vi "ir test.vi"   [LabVIEW 2012, in "Testing.lvrbt"]
uses:
  Testing.lvrbt
  <vilib>/NXT/HiTechnic/HiTechnic Controls/HiTechnic Port.ctl
  <vilib>/NXT/Block Support/NXT_InputPort.ctl
  <vilib>/NXT/Block Support/NXT_ButtonSelector.ctl
  <vilib>/NXT/Dual Mode Library/Sensors/readNXTButton.vi
  <vilib>/NXT/Dual Mode Library/Waits/Wait_Num.vi
  <vilib>/NXT/Dual Mode Library/Display/drawNumber.vi
types:
  T1 = typedef "HiTechnic Port.ctl" = cluster{"Port":T2, "MUX Port":u8}
  T2 = typedef "NXT_InputPort.ctl" = u32
  T3 = typedef "NXT_ButtonSelector.ctl" = u16
  T4 = cluster{"Direction (0-9)":i16, "Signal Strength (Array)":u8[]}
  T5 = typedef "LVHSConnector.ctl" = refnum<class "BrickReference.lvclass">
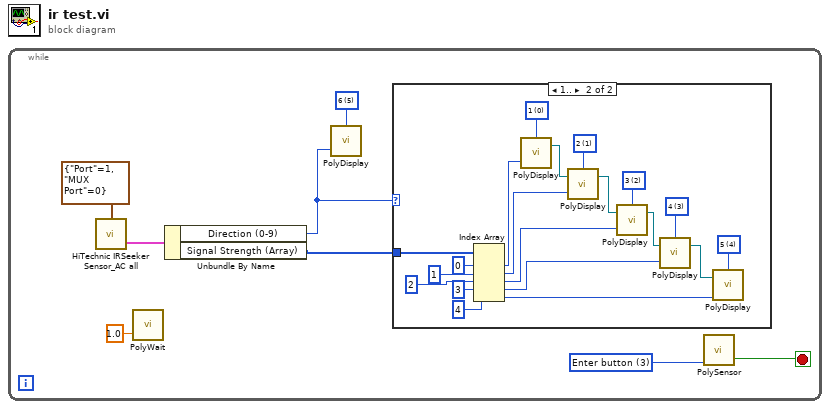
[diagram p0: block diagram]
diagram:
  n1 = while {
    stop <- w4 stop-if-true
    w2 = i16 5 items=["1", "2", "3", "4", "5", "6", "7", "8", "9", "10", "11", "12"] ("Line")
    w5 = T3 3 items=["Enter button"=3, "Left button"=2, "Right button"=1, "Up Button"=4, "Down Button"=5] ("Button (Enter button)")
    n2 = call <vilib>:"HiTechnic IRSeeker Sensor_AC all.vi"("Port/MUX"=T1 {"Port"=1, "MUX Port"=0}) -> ("All Info"=w7:T4)  [unwired: 2 in, 1 out]
    n3 = call-poly <vilib>:"PolyWait.vi"("Time (1 sec)"=sgl 1.0) -> ()  [unwired: 3 in, 1 out]
    n4 = Unbundle By Name(w7) -> ("Direction (0-9)"=w1:i16, "Signal Strength (Array)"=w6:u8[])
    n5 = call-poly <vilib>:"PolyDisplay.vi"("number"=w1, "Line"=w2) -> ()  [unwired: 2 in, 1 out]
    n6 = case shown="1.." w1 {
      tunnel: w6 -> [_ w28]
      frame 0, Default {
      }
      frame 1.. {
        w18 = i16 4 items=["1", "2", "3", "4", "5", "6", "7", "8", "9", "10", "11", "12"] ("Line")
        w19 = i16 3 items=["1", "2", "3", "4", "5", "6", "7", "8", "9", "10", "11", "12"] ("Line")
        w20 = i16 2 items=["1", "2", "3", "4", "5", "6", "7", "8", "9", "10", "11", "12"] ("Line")
        w21 = i16 1 items=["1", "2", "3", "4", "5", "6", "7", "8", "9", "10", "11", "12"] ("Line")
        w26 = i16 0 items=["1", "2", "3", "4", "5", "6", "7", "8", "9", "10", "11", "12"] ("Line")
        n7 = Index Array(array=w28, index #1=0 ("index"), index #2=1 ("index"), index #3=2 ("index"), index #4=3 ("index"), index #5=4 ("index")) -> (element #1=w27:u8, element #2=w25:u8, element #3=w24:u8, element #4=w23:u8, element #5=w22:u8)
        n8 = call-poly <vilib>:"PolyDisplay.vi"("number"=w27, "Line"=w26) -> ("NXT/EV3"=w12:T5)  [unwired: 2 in]
        n9 = call-poly <vilib>:"PolyDisplay.vi"("number"=w25, "NXT/EV3"=w12, "Line"=w21) -> ("NXT/EV3"=w11:T5)  [unwired: 1 in]
        n10 = call-poly <vilib>:"PolyDisplay.vi"("number"=w24, "NXT/EV3"=w11, "Line"=w20) -> ("NXT/EV3"=w10:T5)  [unwired: 1 in]
        n11 = call-poly <vilib>:"PolyDisplay.vi"("number"=w23, "NXT/EV3"=w10, "Line"=w19) -> ("NXT/EV3"=w9:T5)  [unwired: 1 in]
        n12 = call-poly <vilib>:"PolyDisplay.vi"("number"=w22, "NXT/EV3"=w9, "Line"=w18) -> ()  [unwired: 1 in, 1 out]
      }
    }
    n13 = call-poly <vilib>:"PolySensor.vi"("Button (Enter button)"=w5) -> ("Yes/No"=w4:bool)  [unwired: 2 in, 1 out]
  }
